vi "HRM-Stage4-distribute_data.vi"(8 "error in (no error)":errorcluster, 11 "Process data":T1={"Samples size (10)"=10, "Addition signal to remove"=0.0, "Unfiltered wf"={"t0"=timestamp(0 s since 1904-01-01), "dt"=1.0, "Y"=[]}, "Filtered wf"={"t0"=timestamp(0 s since 1904-01-01), "dt"=1.0, "Y"=[]}, "Heart Rate"=0.0, "User Events"={"Signal to remove"=refnum, "Sample size"=refnum, "Filtered wf"=refnum, "Unfiltered wf"=refnum, "Raw wf"=refnum, "Pulse"=refnum, "Stop"=refnum, "Feedback"=refnum, "Run Aqn?"=refnum}}) -> (0 "error out":errorcluster, 3 "Process data out":T1={"Samples size (10)"=10, "Addition signal to remove"=0.0, "Unfiltered wf"={"t0"=timestamp(0 s since 1904-01-01), "dt"=1.0, "Y"=[]}, "Filtered wf"={"t0"=timestamp(0 s since 1904-01-01), "dt"=1.0, "Y"=[]}, "Heart Rate"=0.0, "User Events"={"Signal to remove"=refnum, "Sample size"=refnum, "Filtered wf"=refnum, "Unfiltered wf"=refnum, "Raw wf"=refnum, "Pulse"=refnum, "Stop"=refnum, "Feedback"=refnum, "Run Aqn?"=refnum}})   [LabVIEW 2020]
uses:
  HRM-process-loop_cluster.ctl
  initclose/HRM-Stage4-User_events.ctl
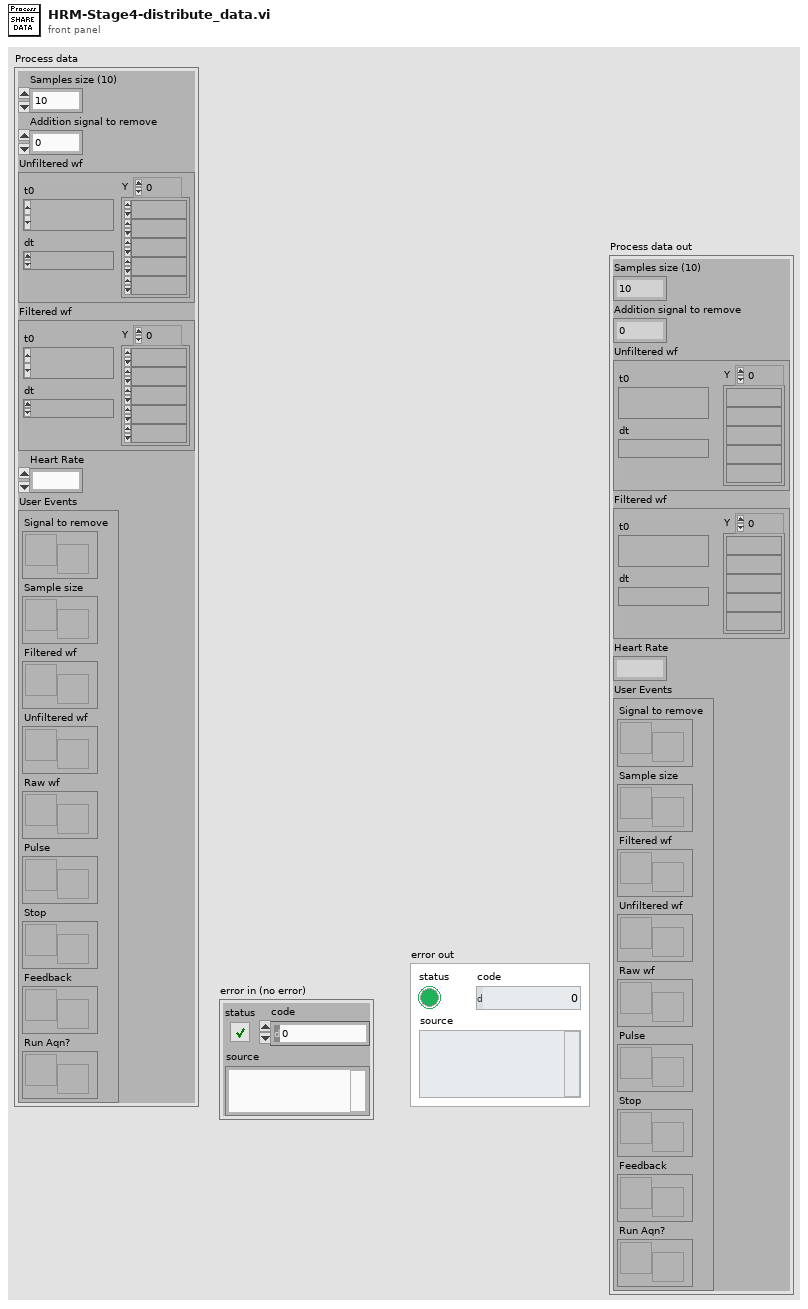
[diagram p1: front panel]
types:
  T1 = typedef "HRM-process-loop_cluster.ctl" = cluster{"Samples size (10)":i32, "Addition signal to remove":dbl, "Unfiltered wf":waveform(dbl), "Filtered wf":waveform(dbl), "Heart Rate":dbl, "User Events":T2}
  T2 = typedef "HRM-Stage4-User_events.ctl" = cluster{"Signal to remove":refnum<user-event>, "Sample size":refnum<user-event>, "Filtered wf":refnum<user-event>, "Unfiltered wf":refnum<user-event>, "Raw wf":refnum<user-event>, "Pulse":refnum<user-event>, "Stop":refnum<user-event>, "Feedback":refnum<user-event>, "Run Aqn?":refnum<user-event>}
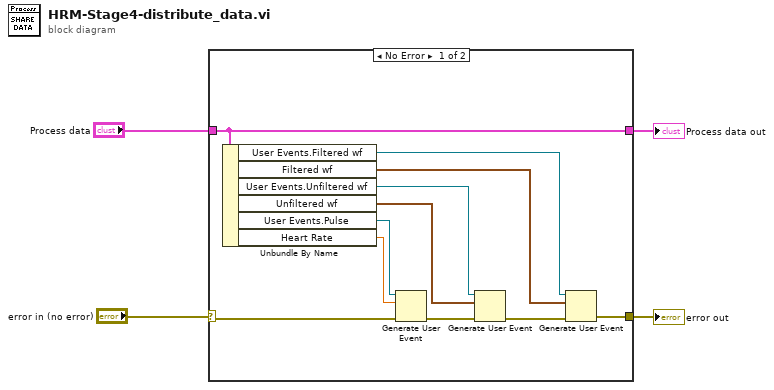
[diagram p0: block diagram]
diagram:
  n1 = case shown="No Error" "error in (no error)" {
    selector: "error in (no error)" -> [w12 w17]
    tunnel: [w13 w17] -> w3
    tunnel: "Process data" -> [w11 w16]
    tunnel: [w11 w16] -> w1
    frame No Error {
      n2 = Unbundle By Name(w11) -> ("User Events.Filtered wf"=w5:refnum<user-event>, "Filtered wf"=w6:waveform(dbl), "User Events.Unfiltered wf"=w7:refnum<user-event>, "Unfiltered wf"=w8:waveform(dbl), "User Events.Pulse"=w9:refnum<user-event>, "Heart Rate"=w10:dbl)
      n3 = Generate User Event(user event=w9, event data cluster=w10, error in=w12) -> (error out=w15:errorcluster)  [unwired: 1 in, 1 out]
      n4 = Generate User Event(user event=w7, event data cluster=w8, error in=w15) -> (error out=w14:errorcluster)  [unwired: 1 in, 1 out]
      n5 = Generate User Event(user event=w5, event data cluster=w6, error in=w14) -> (error out=w13:errorcluster)  [unwired: 1 in, 1 out]
    }
    frame Error {
    }
  }
  "Process data out" <- w1
  "error out" <- w3
